vi "server.Format Client Request (Internal).vi"(8 "error in (no error)":errorcluster, 9 "params":refnum<class "JSON Value.lvclass">, 10 "method":string) -> (0 "error out":errorcluster, 3 "JSON Value out":refnum<class "JSON Value.lvclass">)   [LabVIEW 2016, in "JSONRPC Server.lvclass"]
uses:
  JSONRPC Server.lvclass
  <vilib>/NI/JSON Support for LabVIEW/JSON Value/JSON Value.lvclass
  <vilib>/NI/JSON Support for LabVIEW/JSON Value/New JSON Value/New JSON ({}).vi
  <vilib>/NI/JSON Support for LabVIEW/JSON Value/Object/Insert Value/Insert Value (String).vi
  <vilib>/NI/JSON Support for LabVIEW/JSON Value/Object/Insert Value/Insert Value (Value).vi
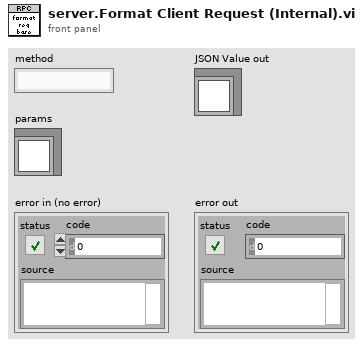
[diagram p1: front panel]
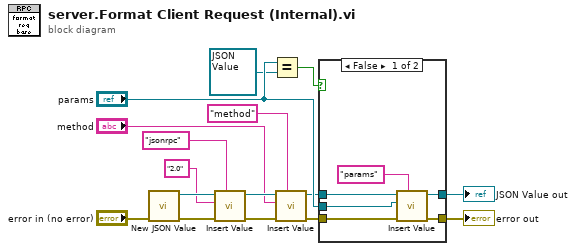
[diagram p0: block diagram]
diagram:
  n1 = call-poly <vilib>:"New JSON Value.vi"("error in (no error)"="error in (no error)") -> ("error out"=w9:errorcluster, "JSON Value out"=w8:refnum<class "JSON Value.lvclass">)  [unwired: 9 in]
  n2 = call-poly <vilib>:"Insert Value.vi"("key"="jsonrpc" ("Name"), "error in (no error)"=w9, "value"="2.0" ("String"), "JSON Value in"=w8) -> ("error out"=w10:errorcluster, "JSON Value out"=w5:refnum<class "JSON Value.lvclass">)  [unwired: 5 in, 1 out]
  n3 = Equal?(x="params", y=refnum<class "JSON Value.lvclass"> refnum ("JSON Value out")) -> (x = y?=w16:bool)
  n4 = call-poly <vilib>:"Insert Value.vi"("key"="method" ("Name"), "error in (no error)"=w10, "value"="method", "JSON Value in"=w5) -> ("error out"=w11:errorcluster, "JSON Value out"=w12:refnum<class "JSON Value.lvclass">)  [unwired: 5 in, 1 out]
  n5 = case shown="False" w16 {
    tunnel: w11 -> [w22 w23]
    tunnel: w12 -> [w19 w24]
    tunnel: [w21 w24] -> w2
    tunnel: [w20 w23] -> w14
    tunnel: "params" -> [w17 _]
    frame False {
      n6 = call-poly <vilib>:"Insert Value.vi"("key"="params" ("Name"), "error in (no error)"=w22, 10:"JSON Value in"=w17, 11:"JSON Value in"=w19) -> ("error out"=w20:errorcluster, "JSON Value out"=w21:refnum<class "JSON Value.lvclass">)  [unwired: 5 in, 1 out]
    }
    frame True {
    }
  }
  "error out" <- w14
  "JSON Value out" <- w2
